vi "shutdown Camera LV.vi"(8 "error in (no error)":errorcluster) -> (0 "error out":errorcluster)   [LabVIEW 2016, in "cameraLibrary.lvlib"]
doc: "Shutdown the camera.\n\nvoid CAMERALIBRARYSHARED_EXPORT shutdownCameraLV();"
uses:
  cameraLibrary.lvlib
  cameraLibrary.dll
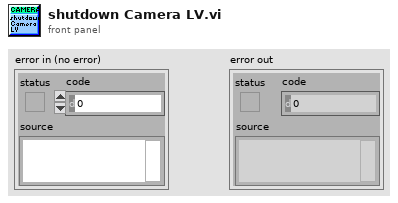
[diagram p1: front panel]
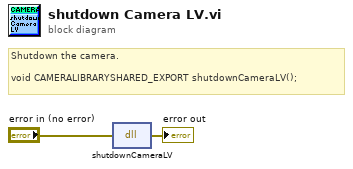
[diagram p0: block diagram]
diagram:
  # "Shutdown the camera.\n\nvoid CAMERALIBRARYSHARED_EXPORT shutdownCameraLV();"
  n1 = dll-call lib="C:/Users/TMM/repos/EXPRES/FEM/FTT/support/Camera Library/cameraLibrary.*" fn="shutdownCameraLV"(error in="error in (no error)") -> (error out=→"error out":errorcluster)  [unwired: 3 in, 1 out]
